vi "Get InitializationVI Node.vi"(8 "error in (no error)":errorcluster, 11 "Project XML Editor in":refnum<class "Project XML Editor.lvclass">) -> (0 "error out":errorcluster, 1 "Found?":bool, 2 "Node ref out":refnum<k20>, 3 "Project XML Editor out":refnum<class "Project XML Editor.lvclass">)   [LabVIEW 2020, in "LVLIBP CD XML Updater.lvlib" / "Project XML Editor.lvclass"]
uses:
  Project XML Editor.lvclass
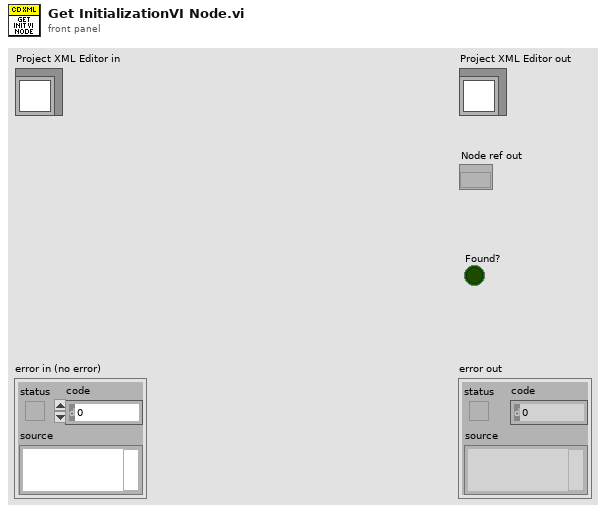
[diagram p1: front panel]
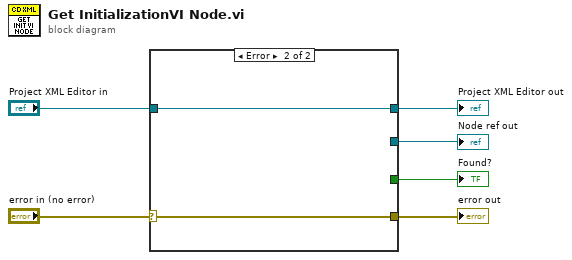
[diagram p0: block diagram]
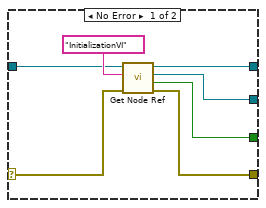
[diagram p2: hidden frame]
diagram:
  n1 = case shown="Error" "error in (no error)" {
    selector: "error in (no error)" -> [w10 w15]
    tunnel: [w9 w15] -> w5
    tunnel: [w11 w14] -> w3
    tunnel: "Project XML Editor in" -> [w12 w14]
    tunnel: [w8 _] -> w2
    tunnel: [w7 _] -> w1
    frame No Error {
      n2 = call "Get Node Ref.vi"("error in (no error)"=w10, "XPath expression"="InitializationVI", "Project XML Editor in"=w12) -> ("error out"=w9:errorcluster, "Found?"=w7:bool, "Node ref out"=w8:refnum<k20>, "Project XML Editor out"=w11:refnum<class "Project XML Editor.lvclass">)  [unwired: 5 in]
    }
    frame Error {
    }
  }
  "error out" <- w5
  "Project XML Editor out" <- w3
  "Node ref out" <- w2
  "Found?" <- w1
